vi "DB_Execute.vi"(8 "error in (no error)":errorcluster, 11 "Humidity":string) -> (0 "error out":errorcluster)   [LabVIEW 2018]
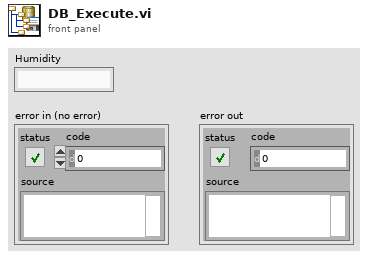
[diagram p1: front panel]
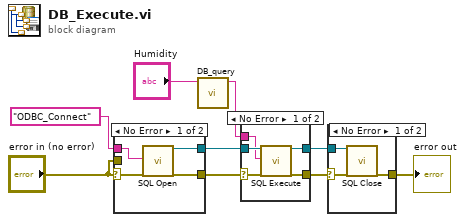
[diagram p0: block diagram]
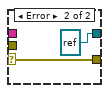
[diagram p4: hidden frame]
diagram:
  n1 = case shown="No Error" "error in (no error)" {
    selector: "error in (no error)" -> [w13 w14]
    tunnel: "error in (no error)" -> [_ _]
    tunnel: [w12 w14] -> w2
    tunnel: [w11 refnum<k7> refnum ("Connection Out")] -> w5
    tunnel: "ODBC_Connect" ("ConnectionString In") -> [w10 _]
    frame No Error {
      n2 = call <vilib>:"SQL Open.vi"("ConnectionString In"=w10, "Error in (no error)"=w13) -> ("Connection Out"=w11:refnum<k7>, "Error out"=w12:errorcluster)  [unwired: 16 in]
    }
    frame Error {
    }
  }
  n3 = call "DB_query.vi"("Humidity"="Humidity") -> ("String"=w9:string)  [unwired: 10 in]
  n4 = case shown="No Error" w2 {
    selector: w2 -> [w20 w21]
    tunnel: [w19 w21] -> w3
    tunnel: w5 -> [w18 w22]
    tunnel: [w17 w22] -> w6
    tunnel: w9 -> [w16 _]
    frame No Error {
      n5 = call <vilib>:"SQL Execute.vi"("Connection In"=w18, "SQL Query"=w16, "Error in (no error)"=w20) -> ("Connection Out"=w17:refnum<k7>, "Error out"=w19:errorcluster)  [unwired: 15 in]
    }
    frame Error {
    }
  }
  n6 = case shown="No Error" w3 {
    selector: w3 -> [w25 w26]
    tunnel: [w24 w26] -> w4
    tunnel: w6 -> [w23 _]
    frame No Error {
      n7 = call <vilib>:"SQL Close.vi"("Connection In"=w23, "Error in (no error)"=w25) -> ("Error out"=w24:errorcluster)  [unwired: 17 in]
    }
    frame Error {
    }
  }
  "error out" <- w4
